vi "FuncImg-Extract single ROI data.vi"(11 "Reordered file paths in ascending file-name order":path[](array[path])) -> (2 "Points per trial":i32, 3 "Data. Y-Axis values":i32[](array[numeric]))   [LabVIEW 2017]
uses:
  <userlib>/My Palettes.lib/Files & paths/Spreadsheet/Read From Spreadsheet File (I64)-Mod.vi
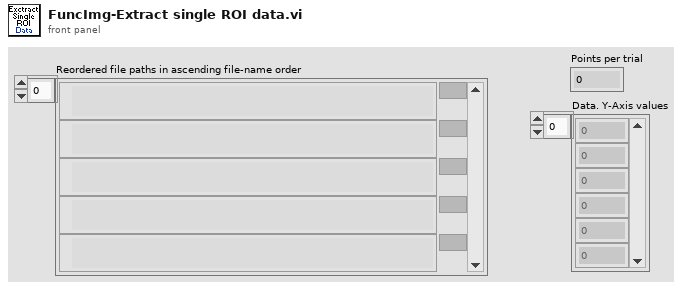
[diagram p1: front panel]
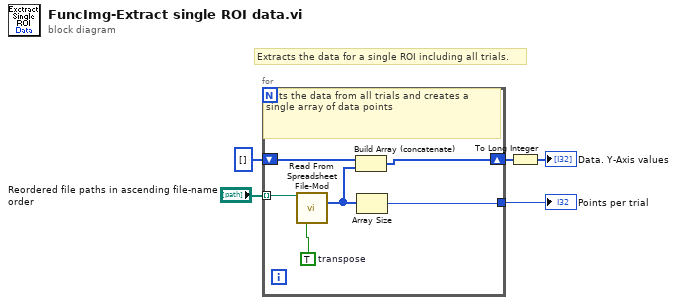
[diagram p0: block diagram]
diagram:
  # "Extracts the data for a single ROI including all trials."
  n1 = for {
    tunnel: "Reordered file paths in ascending file-name order" -> [w6] mode=indexing
    shift-right: [w11] -> w4
    shift-left: i64[] [] -> [w8]
    tunnel: [w10] -> w2
    w9 = TRUE  # transpose
    # "Gets the data from all trials and creates a single array of data points"
    n2 = call-poly <userlib>:"Read From Spreadsheet File-Mod.vi"("file path (dialog if empty)"=w6, "transpose (no:F)"=w9) -> ("first row"=w7:i64[])  [unwired: 8 in, 5 out]
    n3 = Build Array (concatenate)(w8, w7) -> (w11:i64[])
    n4 = Array Size(array=w7) -> (size(s)=w10:i32)
  }
  "Points per trial" <- w2
  n5 = To Long Integer(number=w4) -> (32bit integer=→"Data. Y-Axis values":i32[])
